vi "Test Mic Corr Curve.vi"() -> ()   [LabVIEW 2015]
panel:
  in  "Mic Corr":path
  out "XY Graph":cluster{"Frequency (Hz)":dbl[], "Mag":dbl[]}[](graph)
  in  "PTC":path
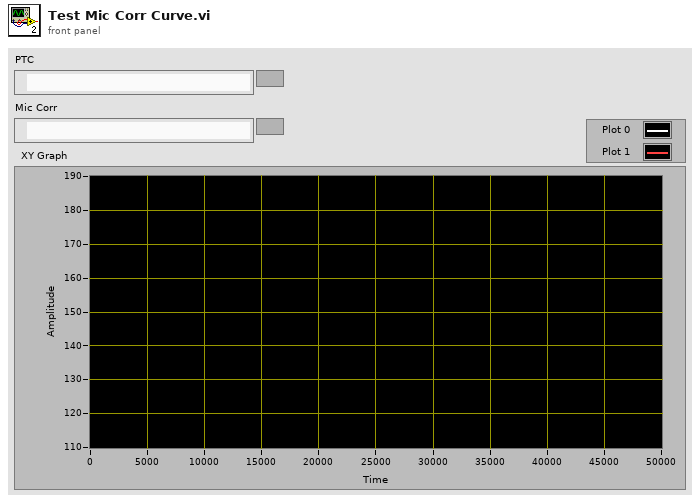
[diagram p1: front panel]
types:
  T1 = cluster{"Frequency out":dbl[], "PTC Mag out":dbl[]}
  T2 = cluster{"Frequency out":dbl[], "PTC Mag out":dbl[]}[]
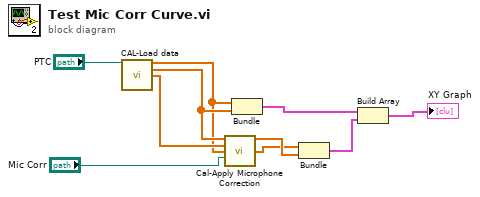
[diagram p0: block diagram]
diagram:
  n1 = call "CAL-Load data.vi"("user path"="PTC") -> ("Frequency (Hz)"=w6:dbl[], "Mag"=w8:dbl[], "Phase"=w7:dbl[])  [unwired: 7 in, 5 out]
  n2 = call "Cal-Apply Microphone Correction.vi"("PTC Mag in"=w8, "PTC Phase in"=w7, "Frequency in"=w6, "Correction curve"="Mic Corr") -> ("PTC Mag out"=w5:dbl[], "Frequency out"=w2:dbl[])  [unwired: 8 in, 2 out]
  n3 = Bundle("Frequency (Hz)"=w6, "Mag"=w8) -> (w9:cluster{"Frequency (Hz)":dbl[], "Mag":dbl[]})  [unwired: 1 in]
  n4 = Bundle("Frequency out"=w2, "PTC Mag out"=w5) -> (w3:T1)  [unwired: 1 in]
  n5 = Build Array(w9, w3) -> (→"XY Graph":T2)
